vi "Main.vi"() -> ()   [LabVIEW 2016]
panel:
  in  "Changelog":string="Line Trace System \nWabco Polska\nMaciej Szupienko\n---------------------------------------------------------------------------------------------------------\nTODO:\n- test cache & export\n- better error handling for database loop\n- get product_component processStepResultId before exporting to DB (not sure)\n---------------------------------------------------------------------------------------------------------\n\nv0.8.5b (2018-08-02)\n- bugfix in TDMS file race condition in write (cache) & read (database)\n- write tdms file in temp folder, when it is written move to correct incoming folder\n\nv0.8.4b (2017-09-26)\n- correct tables position & size at GUI\n\nv0.8.3b (2017-09-20)\n- improve event logs\n- cache thread loop\n\nv0.8.2b (2017-09-15) - not finished\n-  create thread for cache for each process step to avoid file conflict errors\n\nv0.8.1b (2017-09-13)\n-  further cache optimization\n\nv0.8.0b (2017-09-12)\n-  change the cache from one common file per station into multiple small files per product (station/ref/serial)\n- cover product component information in file name\n- create one folder per station for the results\n\nv0.7.5b (2017-09-11)\n- correct error display\n- add filename filter in history gui to find a product result file\n- optimize reading cache files\n- mark as exported at once (opening file takes most of time)\n- add property Pos to use as offset for reading ExportTS table\n\nv0.7.4b (2017-09-08)\n- correct export product/component to database\n- event log viewer\n- correct product viewer\n- correct product tdms files status update\n\nv0.7.3b (2017-09-07)\n- correct exporting cache to DB (not working perfectly yet)\n- continue with line simulator\n- add buffer for cache status\n- add more position in status table\n\nv0.7.2b (2017-09-06)\n- setup GUI for configuring variants\n- correct disconnection of the database clients (prevent db client crash)\n\nv0.7.1b (2017-08-29)\n- correct check previuos station status in database (the same way as in cache)\n- add simulator for Changeover (add NewData and CheckStatus funcitonality)\n- add event logs for cache & database\n\nv0.7.0b (2017-08-28)\n- DB variant sets (2d array for variants/stations defining Prev & This Systems)\n- check previous stations (if 2 stations check for different process/variants - first for product, second for component, both has to be OK)\n- simplify the way of handling systemIDs (Database.Cache.Identify.vi)\n- add Process.Begin/End flags into DB.ini file in order to begin/end process result\n\nv0.6.13b (2017-08-25)\n- 16 db clients (+1)\n- corrections in DUT TDMS result files\n- define process in proda (to be modified)\n\nv0.6.12b (2017-08-24)\n- correct DUT TDMS result status\n- add history screen for DUT results\n\nv0.6.11b (2017-08-24)\n- update DUT TDMS result status\n\nv0.6.10b (2017-08-23)\n- correct loop indexing condition in database GetPrevStatus, GetThisStatus VIs\n- correct channel name in cache ComponentGet & Find VIs\n- add cache DUT TDMS file creation for each product\n\nv0.6.9b (2017-08-18)\n- speed up connection to proda (reentrant connect VI)\n- add station ID column to status table in MainGUI\n- ignore connection error in database handler\n- minor changes in ProdaConfigurator to simplify adding new elements\n- correct MarkExported vi\n\nv0.6.8b (2017-08-18)\n- connect missing Ref in Database-Changeover.vi and Database.Cache.NewData.vi\n- correct formatting strings while reading/writing from/to PLC\n- correct writing float values to PLC\n- correct indexing array in PLC.ReadPLCData.vi\n- write to PLC large portion of data with packages\n\nv0.6.7b (2017-08-17)\n- add and correct CacheInit in AppInit\n- remove ProdaNGInit and ProdaNGExit from AppInit and AppClose (already done in DatabaseHandler)\n- correct Database.Changeover\n- correct Database constructor action (setup method)\n- correct Toolkit for Ini Files (read/write array  to ini file: empty string = empty array)\n- update status table at MainGUI\n- correct initialization of VariantPath in AppInit\n- add StatusGUI table at MainGUI\n- add new top bar status fields for DB & PLC\n- test configuration .dat files\n\nv0.6.6b (2017-08-12)\n- export prod comp list from cache to DB\n- service mode with status (-3)\n\nv0.6.5b (2017-08-11)\n- database handler to choose which data to export (in sequence) and to reconnect all loops at once if dll failed\n\nv0.6.4b (2017-08-10)\n- check prod status\n\nv0.6.3b (2017-08-09)\n- check prod status\n- changeover done (not tested)\n- write to single tdms file per station\n- write prod-comp info to different tdms file\n\nv0.6.2b (2017-08-07)\n- check exist status\n- correct PLC clusters\n\nv0.6.1b (2017-08-03)\n- get prev station status (not ready yet)\n- change name of database thread\n\nv0.6.0b (2017-08-02)\n- proda data cache started (not ready yet)\n\nv0.5 (2017-05-24)\n- autoscaling of the main gui\n- add changeover\n\nv0.4 (2017-05-23)\n- downgrade to LV 2015\n\nv0.3 (2017-05-04)\n- correct proda disconnection\n\nv0.2 (2017-04-27)\n- extend to 3 PLCs and 3 DBs\n\nv0.1 (2017-03-29)\n- demo for supplier" caption="MAKE CURRENT VALUE DEFAULT!!!"
  # "VERSION UNDER TEST !!!"
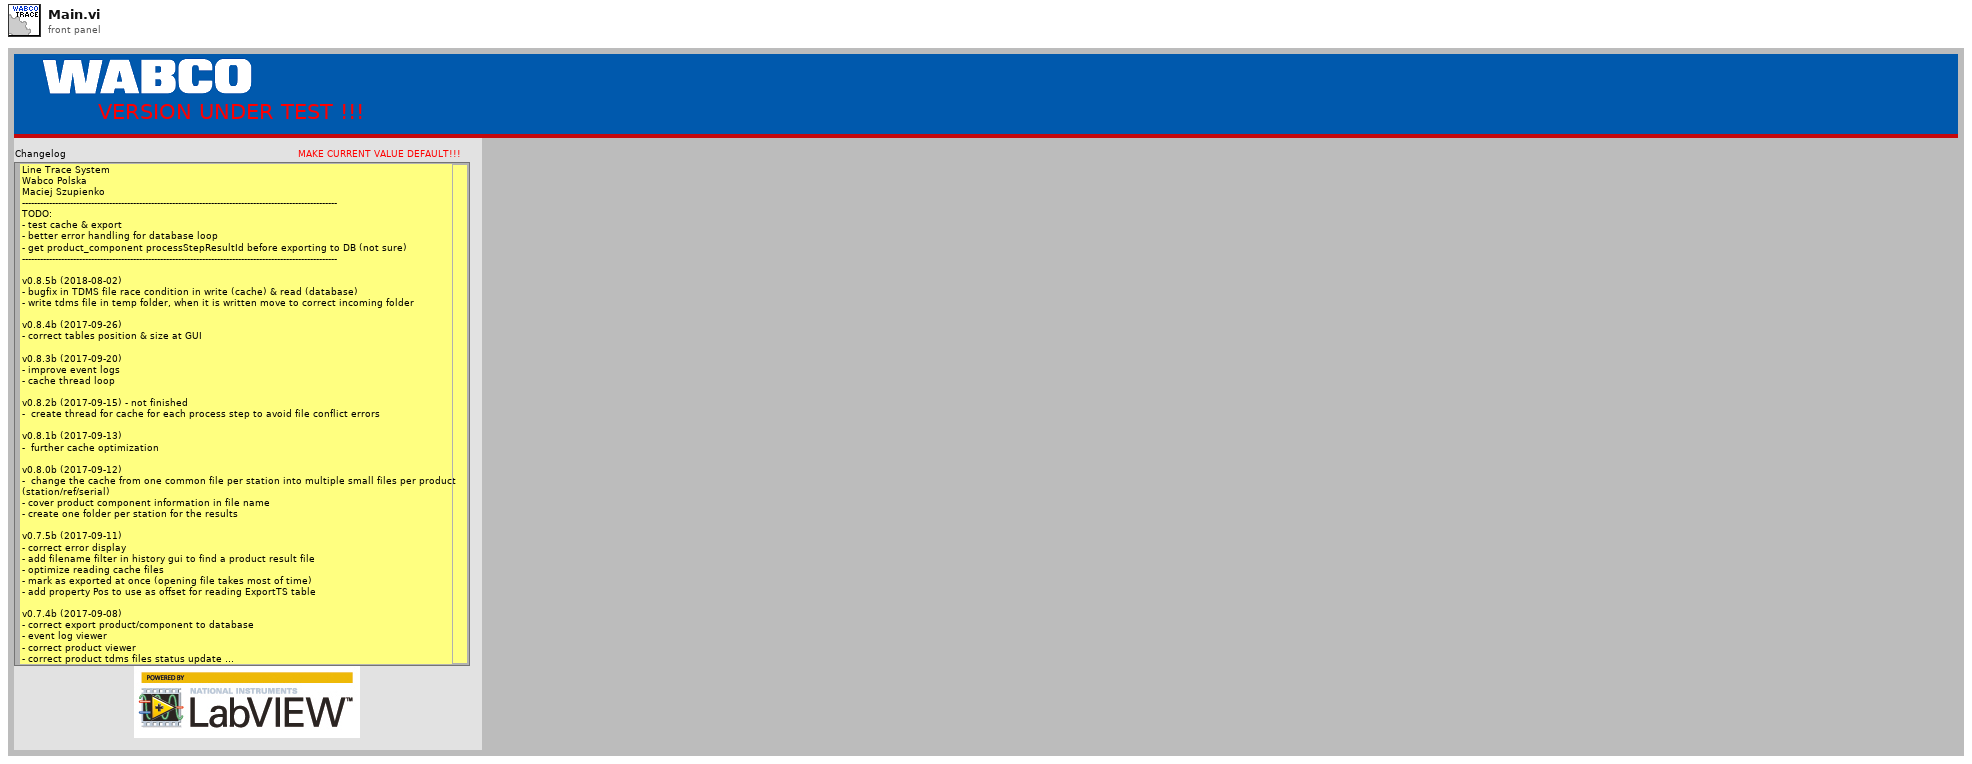
[diagram p1: front panel]
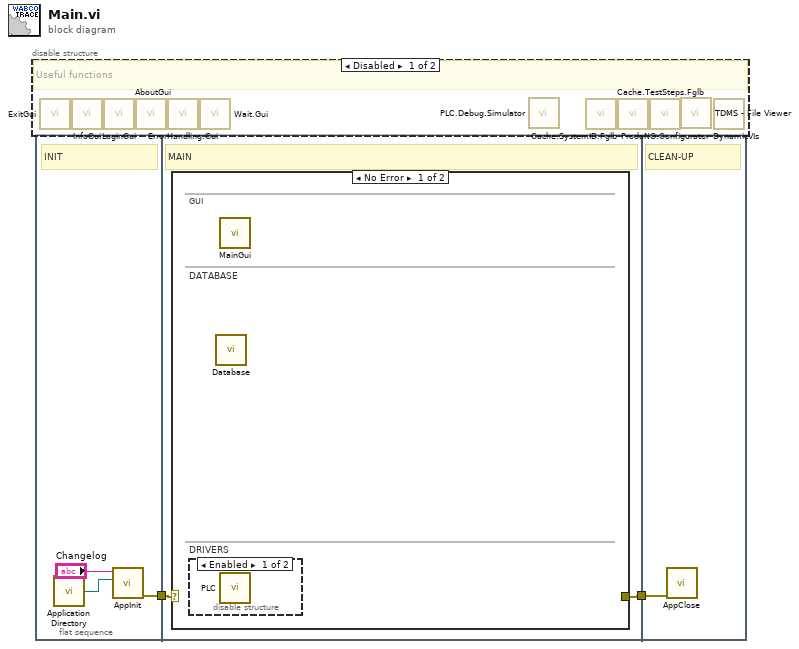
[diagram p0: block diagram]
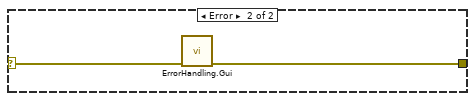
[diagram p3: hidden frame]
diagram:
  n1 = disable-structure shown="Disabled" {
    frame Disabled {
      # "Useful functions"
      n2 = call "ExitGui.vi"() -> ()  [unwired: 10 in, 2 out]
      n3 = call "InfoGui.vi"() -> ()  [unwired: 11 in, 1 out]
      n4 = call "LoginGui.vi"() -> ()  [unwired: 11 in, 1 out]
      n5 = call "AboutGui.vi"() -> ()  [unwired: 12 in]
      n6 = call "ErrorHandling.Gui.vi"() -> ()  [unwired: 10 in, 2 out]
      n7 = call "Wait.Gui.vi"() -> ()  [unwired: 12 in]
      n8 = call "PLC.Debug.Simulator.vi"() -> ()  [unwired: 12 in]
      n9 = call "Cache.SystemID.Fglb.vi"() -> ()  [unwired: 9 in, 3 out]
      n10 = call "Cache.TestSteps.Fglb.vi"() -> ()  [unwired: 8 in, 4 out]
      n11 = call "ProdaNG.Configurator.vi"() -> ()  [unwired: 12 in]
      n12 = call <vilib>:"TDMS - File Viewer.vi"() -> ()  [unwired: 6 in, 2 out]
      n13 = call "DynamicVIs.vi"() -> ()  [unwired: 12 in]
    }
    frame Enabled {
    }
  }
  n14 = flat-sequence {
    tunnel: [w4] -> w2
    tunnel: w2 -> [w7]
    tunnel: [w6] -> w1
    tunnel: w1 -> [w10]
    frame #0 {
      # "INIT"
      n15 = call <vilib>:"Application Directory.vi"() -> ("Application Directory"=w3:path)
      n16 = call "AppInit.vi"("path"=w3, "Changelog"="Changelog") -> ("error out"=w4:errorcluster)  [unwired: 9 in]
    }
    frame #1 {
      # "MAIN"
      n17 = case shown="No Error" w7 {
        selector: w7 -> [_ w9]
        tunnel: [_ w8] -> w6
        frame No Error {
          # "GUI"
          # "DATABASE"
          # "DRIVERS"
          n18 = disable-structure shown="Enabled" {
            frame Enabled {
              n19 = call "PLC.vi"() -> ()  [unwired: 12 in]
            }
            frame Disabled {
            }
          }
          n20 = call "Database.vi"() -> ()  [unwired: 12 in]
          n21 = call "MainGui.vi"() -> ()  [unwired: 1 in]
        }
        frame Error {
          n22 = call "ErrorHandling.Gui.vi"("error in (no error)"=w9) -> ("error out"=w8:errorcluster)  [unwired: 9 in, 1 out]
        }
      }
    }
    frame #2 {
      # "CLEAN-UP"
      n23 = call "AppClose.vi"("error in (no error)"=w10) -> ()  [unwired: 11 in]
    }
  }
